vi "DisplayJson.vi"(11 "JSON String In":string="[{\"version\":\"1.0.0\",\"header\":{\"creationDate\":\"2022-06-03T00:00:00\",\"remarks\":\"\",\"serialNumber\":\"98172\",\"productNumber\":\"123021.1804\",\"productType\":\"PAA-9L\",\"pressureType\":2,\"productSeries\":\"9L\",\"compensatedTemperatureRange\":{\"min\":-10.0,\"max\":80.0,\"unit\":4},\"compensatedPressureRange\":{\"min\":0.0,\"max\":0.35,\"unit\":3},\"electricSupply\":{\"magnitude\":1.0,\"unit\":18},\"orderNumber\":9990266,\"orderPosition\":3,\"orderTargetDispatchDate\":\"2022-06-02T00:00:00+00:00\",\"customerName\":\"DemoData Inc.\",\"customerNumber\":12345678,\"customerOrderNumber\":\"Cust-9990266-123\",\"customerReferenceNumber\":\"\",\"customerProductT...") -> ()   [LabVIEW 2017] (continued)
\"unit\":4},\"supply\":{\"magnitude\":1.0,\"unit\":18}},\"raw\":{\"signal\":{\"magnitude\":16.118017703,\"unit\":22},\"bridgeResistance\":{\"magnitude\":3275.904706,\"unit\":28}},\"compensated\":{\"mathematicalModels\":{\"MM0123\":{\"pressure\":{\"output\":{\"magnitude\":0.0300104,\"unit\":3},\"error\":{\"magnitude\":0.00331228,\"unit\":7}},\"temperature\":{\"output\":{\"magnitude\":-10.8322,\"unit\":4},\"error\":{\"magnitude\":-0.10352768,\"unit\":4}}}}}},{\"reference\":\"F_12300_XX_0000098765\",\"environmentTarget\":{\"pressure\":{\"magnitude\":0.11,\"unit\":3},\"temperature\":{\"magnitude\":-10.0,\"unit\":4}},\"environment\":{\"pressure\":{\"magnitude\":0.110001,\"unit\":3},\"temperature\":{\"magnitude\":-10.7286,\"unit\":4},\"supply\":{\"magnitude\":1.0,\"unit\":18}},\"raw\":{\"signal\":{\"magnitude\":27.050815771,\"unit\":22},\"bridgeResistance\":{\"magnitude\":3271.7296615,\"unit\":28}},\"compensated\":{\"mathematicalModels\":{\"MM0123\":{\"pressure\":{\"output\":{\"magnitude\":0.109974,\"unit\":3},\"error\":{\"magnitude\":-0.0076162767,\"unit\":7}},\"temperature\":{\"output\":{\"magnitude\":-10.839,\"unit\":4},\"error\":{\"magnitude\":-0.11034124,\"unit\":4}}}}}},{\"reference\":\"F_12300_XX_0000098765\",\"environmentTarget\":{\"pressure\":{\"magnitude\":0.19,\"unit\":3},\"temperature\":{\"magnitude\":-10.0,\"unit\":4}},\"environment\":{\"pressure\":{\"magnitude\":0.190006,\"unit\":3},\"temperature\":{\"magnitude\":-10.7286,\"unit\":4},\"supply\":{\"magnitude\":1.0,\"unit\":18}},\"raw\":{\"signal\":{\"magnitude\":37.952972523,\"unit\":22},\"bridgeResistance\":{\"magnitude\":3267.7437326,\"unit\":28}},\"compensated\":{\"mathematicalModels\":{\"MM0123\":{\"pressure\":{\"output\":{\"magnitude\":0.190012,\"unit\":3},\"error\":{\"magnitude\":0.0016039999,\"unit\":7}},\"temperature\":{\"output\":{\"magnitude\":-10.8327,\"unit\":4},\"error\":{\"magnitude\":-0.10406948,\"unit\":4}}}}}},{\"reference\":\"F_12300_XX_0000098765\",\"environmentTarget\":{\"pressure\":{\"magnitude\":0.27,\"unit\":3},\"temperature\":{\"magnitude\":-10.0,\"unit\":4}},\"environment\":{\"pressure\":{\"magnitude\":0.270002,\"unit\":3},\"temperature\":{\"magnitude\":-10.7286,\"unit\":4},\"supply\":{\"magnitude\":1.0,\"unit\":18}},\"raw\":{\"signal\":{\"magnitude\":48.811226671,\"unit\":22},\"bridgeResistance\":{\"magnitude\":3263.8401462,\"unit\":28}},\"compensated\":{\"mathematicalModels\":{\"MM0123\":{\"pressure\":{\"output\":{\"magnitude\":0.270032,\"unit\":3},\"error\":{\"magnitude\":0.0086056558,\"unit\":7}},\"temperature\":{\"output\":{\"magnitude\":-10.8305,\"unit\":4},\"error\":{\"magnitude\":-0.10182691,\"unit\":4}}}}}},{\"reference\":\"F_12300_XX_0000098765\",\"environmentTarget\":{\"pressure\":{\"magnitude\":0.35,\"unit\":3},\"temperature\":{\"magnitude\":-10.0,\"unit\":4}},\"environment\":{\"pressure\":{\"magnitude\":0.350003,\"unit\":3},\"temperature\":{\"magnitude\":-10.7286,\"unit\":4},\"supply\":{\"magnitude\":1.0,\"unit\":18}},\"raw\":{\"signal\":{\"magnitude\":59.620114048,\"unit\":22},\"bridgeResistance\":{\"magnitude\":3259.9998996,\"unit\":28}},\"compensated\":{\"mathematicalModels\":{\"MM0123\":{\"pressure\":{\"output\":{\"magnitude\":0.349997,\"unit\":3},\"error\":{\"magnitude\":-0.0016426142,\"unit\":7}},\"temperature\":{\"output\":{\"magnitude\":-10.8357,\"unit\":4},\"error\":{\"magnitude\":-0.10710598,\"unit\":4}}}}}},{\"reference\":\"F_12300_XX_0000098765\",\"environmentTarget\":{\"pressure\":{\"magnitude\":0.03,\"unit\":3},\"temperature\":{\"magnitude\":0.0,\"unit\":4}},\"environment\":{\"pressure\":{\"magnitude\":0.0299997,\"unit\":3},\"temperature\":{\"magnitude\":-0.629962,\"unit\":4},\"supply\":{\"magnitude\":1.0,\"unit\":18}},\"raw\":{\"signal\":{\"magnitude\":16.568926387,\"unit\":22},\"bridgeResistance\":{\"magnitude\":3345.7360415,\"unit\":28}},\"compensated\":{\"mathematicalModels\":{\"MM0123\":{\"pressure\":{\"output\":{\"magnitude\":0.0300107,\"unit\":3},\"error\":{\"magnitude\":0.0031346511,\"unit\":7}},\"temperature\":{\"output\":{\"magnitude\":-0.744773,\"unit\":4},\"error\":{\"magnitude\":-0.11481098,\"unit\":4}}}}}},{\"reference\":\"F_12300_XX_0000098765\",\"environmentTarget\":{\"pressure\":{\"magnitude\":0.11,\"unit\":3},\"temperature\":{\"magnitude\":0.0,\"unit\":4}},\"environment\":{\"pressure\":{\"magnitude\":0.109998,\"unit\":3},\"temperature\":{\"magnitude\":-0.629962,\"unit\":4},\"supply\":{\"magnitude\":1.0,\"unit\":18}},\"raw\":{\"signal\":{\"magnitude\":27.469706317,\"unit\":22},\"bridgeResistance\":{\"magnitude\":3341.6261347,\"unit\":28}},\"compensated\":{\"mathematicalModels\":{\"MM0123\":{\"pressure\":{\"output\":{\"magnitude\":0.109974,\"unit\":3},\"error\":{\"magnitude\":-0.0069126471,\"unit\":7}},\"temperature\":{\"output\":{\"magnitude\":-0.743796,\"unit\":4},\"error\":{\"magnitude\":-0.11383453,\"unit\":4}}}}}},{\"reference\":\"F_12300_XX_0000098765\",\"environmentTarget\":{\"pressure\":{\"magnitude\":0.19,\"unit\":3},\"temperature\":{\"magnitude\":0.0,\"unit\":4}},\"environment\":{\"pressure\":{\"magnitude\":0.190003,\"unit\":3},\"temperature\":{\"magnitude\":-0.629962,\"unit\":4},\"supply\":{\"magnitude\":1.0,\"unit\":18}},\"raw\":{\"signal\":{\"magnitude\":38.339532672,\"unit\":22},\"bridgeResistance\":{\"magnitude\":3337.5825723,\"unit\":28}},\"compensated\":{\"mathematicalModels\":{\"MM0123\":{\"pressure\":{\"output\":{\"magnitude\":0.189998,\"unit\":3},\"error\":{\"magnitude\":-0.0014345835,\"unit\":7}},\"temperature\":{\"output\":{\"magnitude\":-0.746189,\"unit\":4},\"error\":{\"magnitude\":-0.11622639,\"unit\":4}}}}}},{\"reference\":\"F_12300_XX_0000098765\",\"environmentTarget\":{\"pressure\":{\"magnitude\":0.27,\"unit\":3},\"temperature\":{\"magnitude\":0.0,\"unit\":4}},\"environment\":{\"pressure\":{\"magnitude\":0.269999,\"unit\":3},\"temperature\":{\"magnitude\":-0.629962,\"unit\":4},\"supply\":{\"magnitude\":1.0,\"unit\":18}},\"raw\":{\"signal\":{\"magnitude\":49.167977875,\"unit\":22},\"bridgeResistance\":{\"magnitude\":3333.6130156,\"unit\":28}},\"compensated\":{\"mathematicalModels\":{\"MM0123\":{\"pressure\":{\"output\":{\"magnitude\":0.270007,\"unit\":3},\"error\":{\"magnitude\":0.0023560799,\"unit\":7}},\"temperature\":{\"output\":{\"magnitude\":-0.751685,\"unit\":4},\"error\":{\"magnitude\":-0.12172338,\"unit\":4}}}}}},{\"reference\":\"F_12300_XX_0000098765\",\"environmentTarget\":{\"pressure\":{\"magnitude\":0.35,\"unit\":3},\"temperature\":{\"magnitude\":0.0,\"unit\":4}},\"environment\":{\"pressure\":{\"magnitude\":0.350005,\"unit\":3},\"temperature\":{\"magnitude\":-0.629962,\"unit\":4},\"supply\":{\"magnitude\":1.0,\"unit\":18}},\"raw\":{\"signal\":{\"magnitude\":59.952257941,\"unit\":22},\"bridgeResistance\":{\"magnitude\":3329.770464,\"unit\":28}},\"compensated\":{\"mathematicalModels\":{\"MM0123\":{\"pressure\":{\"output\":{\"magnitude\":0.349979,\"unit\":3},\"error\":{\"magnitude\":-0.0073028693,\"unit\":7}},\"temperature\":{\"output\":{\"magnitude\":-0.753307,\"unit\":4},\"error\":{\"magnitude\":-0.12334541,\"unit\":4}}}}}},{\"reference\":\"F_12300_XX_0000098765\",\"environmentTarget\":{\"pressure\":{\"magnitude\":0.03,\"unit\":3},\"temperature\":{\"magnitude\":20.0,\"unit\":4}},\"environment\":{\"pressure\":{\"magnitude\":0.0300032,\"unit\":3},\"temperature\":{\"magnitude\":19.5509,\"unit\":4},\"supply\":{\"magnitude\":1.0,\"unit\":18}},\"raw\":{\"signal\":{\"magnitude\":17.508789568,\"unit\":22},\"bridgeResistance\":{\"magnitude\":3502.485602,\"unit\":28}},\"compensated\":{\"mathematicalModels\":{\"MM0123\":{\"pressure\":{\"output\":{\"magnitude\":0.0300153,\"unit\":3},\"error\":{\"magnitude\":0.0034436329,\"unit\":7}},\"temperature\":{\"output\":{\"magnitude\":19.5499,\"unit\":4},\"error\":{\"magnitude\":-0.00093978929,\"unit\":4}}}}}},{\"reference\":\"F_12300_XX_0000098765\",\"environmentTarget\":{\"pressure\":{\"magnitude\":0.11,\"unit\":3},\"temperature\":{\"magnitude\":20.0,\"unit\":4}},\"environment\":{\"pressure\":{\"magnitude\":0.109996,\"unit\":3},\"temperature\":{\"magnitude\":19.5509,\"unit\":4},\"supply\":{\"magnitude\":1.0,\"unit\":18}},\"raw\":{\"signal\":{\"magnitude\":28.398706548,\"unit\":22},\"bridgeResistance\":{\"magnitude\":3498.325108,\"unit\":28}},\"compensated\":{\"mathematicalModels\":{\"MM0123\":{\"pressure\":{\"output\":{\"magnitude\":0.109974,\"unit\":3},\"error\":{\"magnitude\":-0.0063104891,\"unit\":7}},\"temperature\":{\"output\":{\"magnitude\":19.5428,\"unit\":4},\"error\":{\"magnitude\":-0.0081190802,\"unit\":4}}}}}},{\"reference\":\"F_12300_XX_0000098765\",\"environmentTarget\":{\"pressure\":{\"magnitude\":0.19,\"unit\":3},\"temperature\":{\"magnitude\":20.0,\"unit\":4}},\"environment\":{\"pressure\":{\"magnitude\":0.189992,\"unit\":3},\"temperature\":{\"magnitude\":19.5509,\"unit\":4},\"supply\":{\"magnitude\":1.0,\"unit\":18}},\"raw\":{\"signal\":{\"magnitude\":39.263123148,\"unit\":22},\"bridgeResistance\":{\"magnitude\":3494.3052236,\"unit\":28}},\"compensated\":{\"mathematicalModels\":{\"MM0123\":{\"pressure\":{\"output\":{\"magnitude\":0.190003,\"unit\":3},\"error\":{\"magnitude\":0.0031341282,\"unit\":7}},\"temperature\":{\"output\":{\"magnitude\":19.5435,\"unit\":4},\"error\":{\"magnitude\":-0.0073409516,\"unit\":4}}}}}},{\"reference\":\"F_12300_XX_0000098765\",\"environmentTarget\":{\"pressure\":{\"magnitude\":0.27,\"unit\":3},\"temperature\":{\"magnitude\":20.0,\"unit\":4}},\"environment\":{\"pressure\":{\"magnitude\":0.269993,\"unit\":3},\"temperature\":{\"magnitude\":19.5509,\"unit\":4},\"supply\":{\"magnitude\":1.0,\"unit\":18}},\"raw\":{\"signal\":{\"magnitude\":50.090798002,\"unit\":22},\"bridgeResistance\":{\"magnitude\":3490.3161774,\"unit\":28}},\"compensated\":{\"mathematicalModels\":{\"MM0123\":{\"pressure\":{\"output\":{\"magnitude\":0.270025,\"unit\":3},\"error\":{\"magnitude\":0.0091306696,\"unit\":7}},\"temperature\":{\"output\":{\"magnitude\":19.5384,\"unit\":4},\"error\":{\"magnitude\":-0.012497416,\"unit\":4}}}}}},{\"reference\":\"F_12300_XX_0000098765\",\"environmentTarget\":{\"pressure\":{\"magnitude\":0.35,\"unit\":3},\"temperature\":{\"magnitude\":20.0,\"unit\":4}},\"environment\":{\"pressure\":{\"magnitude\":0.350012,\"unit\":3},\"temperature\":{\"magnitude\":19.5509,\"unit\":4},\"supply\":{\"magnitude\":1.0,\"unit\":18}},\"raw\":{\"signal\":{\"magnitude\":60.879181622,\"unit\":22},\"bridgeResistance\":{\"magnitude\":3486.4490777,\"unit\":28}},\"compensated\":{\"mathematicalModels\":{\"MM0123\":{\"pressure\":{\"output\":{\"magnitude\":0.350017,\"unit\":3},\"error\":{\"magnitude\":0.0013342798,\"unit\":7}},\"temperature\":{\"output\":{\"magnitude\":19.5381,\"unit\":4},\"error\":{\"magnitude\":-0.012768281,\"unit\":4}}}}}},{\"reference\":\"F_12300_XX_0000098765\",\"environmentTarget\":{\"pressure\":{\"magnitude\":0.03,\"unit\":3},\"temperature\":{\"magnitude\":40.0,\"unit\":4}},\"environment\":{\"pressure\":{\"magnitude\":0.0299978,\"unit\":3},\"temperature\":{\"magnitude\":39.7284,\"unit\":4},\"supply\":{\"magnitude\":1.0,\"unit\":18}},\"raw\":{\"signal\":{\"magnitude\":18.512052925,\"unit\":22},\"bridgeResistance\":{\"magnitude\":3678.2402787,\"unit\":28}},\"compensated\":{\"mathematicalModels\":{\"MM0123\":{\"pressure\":{\"output\":{\"magnitude\":0.0300125,\"unit\":3},\"error\":{\"magnitude\":0.0041964975,\"unit\":7}},\"temperature\":{\"output\":{\"magnitude\":39.7197,\"unit\":4},\"error\":{\"magnitude\":-0.0086930497,\"unit\":4}}}}}},{\"reference\":\"F_12300_XX_0000098765\",\"environmentTarget\":{\"pressure\":{\"magnitude\":0.11,\"unit\":3},\"temperature\":{\"magnitude\":40.0,\"unit\":4}},\"environment\":{\"pressure\":{\"magnitude\":0.110012,\"unit\":3},\"temperature\":{\"magnitude\":39.7284,\"unit\":4},\"supply\":{\"magnitude\":1.0,\"unit\":18}},\"raw\":{\"signal\":{\"magnitude\":29.451517412,\"unit\":22},\"bridgeResistance\":{\"magnitude\":3674.1165555,\"unit\":28}},\"compensated\":{\"mathematicalModels\":{\"MM0123\":{\"pressure\":{\"output\":{\"magnitude\":0.109976,\"unit\":3},\"error\":{\"magnitude\":-0.01022075,\"unit\":7}},\"temperature\":{\"output\":{\"magnitude\":39.7193,\"unit\":4},\"error\":{\"magnitude\":-0.0091078646,\"unit\":4}}}}}},{\"reference\":\"F_12300_XX_0000098765\",\"environmentTarget\":{\"pressure\":{\"magnitude\":0.19,\"unit\":3},\"temperature\":{\"magnitude\":40.0,\"unit\":4}},\"environment\":{\"pressure\":{\"magnitude\":0.190003,\"unit\":3},\"temperature\":{\"magnitude\":39.7284,\"unit\":4},\"supply\":{\"magnitude\":1.0,\"unit\":18}},\"raw\":{\"signal\":{\"magnitude\":40.368344408,\"unit\":22},\"bridgeResistance\":{\"magnitude\":3670.043361,\"unit\":28}},\"compensated\":{\"mathematicalModels\":{\"MM0123\":{\"pressure\":{\"output\":{\"magnitude\":0.190005,\"unit\":3},\"error\":{\"magnitude\":0.00066025861,\"unit\":7}},\"temperature\":{\"output\":{\"magnitude\":39.7172,\"unit\":4},\"error\":{\"magnitude\":-0.01127367,\"unit\":4}}}}}},{\"reference\":\"F_12300_XX_0000098765\",\"environmentTarget\":{\"pressure\":{\"magnitude\":0.27,\"unit\":3},\"temperature\":{\"magnitude\":40.0,\"unit\":4}},\"environment\":{\"pressure\":{\"magnitude\":0.269991,\"unit\":3},\"temperature\":{\"magnitude\":39.7284,\"unit\":4},\"supply\":{\"magnitude\":1.0,\"unit\":18}},\"raw\":{\"signal\":{\"magnitude\":51.249896616,\"unit\":22},\"bridgeResistance\":{\"magnitude\":3666.0556113,\"unit\":28}},\"compensated\":{\"mathematicalModels\":{\"MM0123\":{\"pressure\":{\"output\":{\"magnitude\":0.270006,\"unit\":3},\"error\":{\"magnitude\":0.0043130135,\"unit\":7}},\"temperature\":{\"output\":{\"magnitude\":39.7168,\"unit\":4},\"error\":{\"magnitude\":-0.011660585,\"unit\":4}}}}}},{\"reference\":\"F_12300_XX_0000098765\",\"environmentTarget\":{\"pressure\":{\"magnitude\":0.35,\"unit\":3},\"temperature\":{\"magnitude\":40.0,\"unit\":4}},\"environment\":{\"pressure\":{\"magnitude\":0.350007,\"unit\":3},\"temperature\":{\"magnitude\":39.7284,\"unit\":4},\"supply\":{\"magnitude\":1.0,\"unit\":18}},\"raw\":{\"signal\":{\"magnitude\":62.096595353,\"unit\":22},\"bridgeResistance\":{\"magnitude\":3662.1121149,\"unit\":28}},\"compensated\":{\"mathematicalModels\":{\"MM0123\":{\"pressure\":{\"output\":{\"magnitude\":0.349984,\"unit\":3},\"error\":{\"magnitude\":-0.006660769,\"unit\":7}},\"temperature\":{\"output\":{\"magnitude\":39.7132,\"unit\":4},\"error\":{\"magnitude\":-0.015214193,\"unit\":4}}}}}},{\"reference\":\"F_12300_XX_0000098765\",\"environmentTarget\":{\"pressure\":{\"magnitude\":0.03,\"unit\":3},\"temperature\":{\"magnitude\":60.0,\"unit\":4}},\"environment\":{\"pressure\":{\"magnitude\":0.0299911,\"unit\":3},\"temperature\":{\"magnitude\":59.8651,\"unit\":4},\"supply\":{\"magnitude\":1.0,\"unit\":18}},\"raw\":{\"signal\":{\"magnitude\":19.614878521,\"unit\":22},\"bridgeResistance\":{\"magnitude\":3870.4360415,\"unit\":28}},\"compensated\":{\"mathematicalModels\":{\"MM0123\":{\"pressure\":{\"output\":{\"magnitude\":0.0300063,\"unit\":3},\"error\":{\"magnitude\":0.0043445952,\"unit\":7}},\"temperature\":{\"output\":{\"magnitude\":59.9283,\"unit\":4},\"error\":{\"magnitude\":0.063173095,\"unit\":4}}}}}},{\"reference\":\"F_12300_XX_0000098765\",\"environmentTarget\":{\"pressure\":{\"magnitude\":0.11,\"unit\":3},\"temperature\":{\"magnitude\":60.0,\"unit\":4}},\"environment\":{\"pressure\":{\"magnitude\":0.11,\"unit\":3},\"temperature\":{\"magnitude\":59.8651,\"unit\":4},\"supply\":{\"magnitude\":1.0,\"unit\":18}},\"raw\":{\"signal\":{\"magnitude\":30.638429504,\"unit\":22},\"bridgeResistance\":{\"magnitude\":3866.2610003,\"unit\":28}},\"compensated\":{\"mathematicalModels\":{\"MM0123\":{\"pressure\":{\"output\":{\"magnitude\":0.10997,\"unit\":3},\"error\":{\"magnitude\":-0.0086978031,\"unit\":7}},\"temperature\":{\"output\":{\"magnitude\":59.9299,\"unit\":4},\"error\":{\"magnitude\":0.06477835,\"unit\":4}}}}}},{\"reference\":\"F_12300_XX_0000098765\",\"environmentTarget\":{\"pressure\":{\"magnitude\":0.19,\"unit\":3},\"temperature\":{\"magnitude\":60.0,\"unit\":4}},\"environment\":{\"pressure\":{\"magnitude\":0.189995,\"unit\":3},\"temperature\":{\"magnitude\":59.8651,\"unit\":4},\"supply\":{\"magnitude\":1.0,\"unit\":18}},\"raw\":{\"signal\":{\"magnitude\":41.64509949,\"unit\":22},\"bridgeResistance\":{\"magnitude\":3862.1495484,\"unit\":28}},\"compensated\":{\"mathematicalModels\":{\"MM0123\":{\"pressure\":{\"output\":{\"magnitude\":0.190003,\"unit\":3},\"error\":{\"magnitude\":0.00236892,\"unit\":7}},\"temperature\":{\"output\":{\"magnitude\":59.9328,\"unit\":4},\"error\":{\"magnitude\":0.067646361,\"unit\":4}}}}}},{\"reference\":\"F_12300_XX_0000098765\",\"environmentTarget\":{\"pressure\":{\"magnitude\":0.27,\"unit\":3},\"temperature\":{\"magnitude\":60.0,\"unit\":4}},\"environment\":{\"pressure\":{\"magnitude\":0.270008,\"unit\":3},\"temperature\":{\"magnitude\":59.8651,\"unit\":4},\"supply\":{\"magnitude\":1.0,\"unit\":18}},\"raw\":{\"signal\":{\"magnitude\":52.624237436,\"unit\":22},\"bridgeResistance\":{\"magnitude\":3858.0534892,\"unit\":28}},\"compensated\":{\"mathematicalModels\":{\"MM0123\":{\"pressure\":{\"output\":{\"magnitude\":0.270034,\"unit\":3},\"error\":{\"magnitude\":0.007359755,\"unit\":7}},\"temperature\":{\"output\":{\"magnitude\":59.9315,\"unit\":4},\"error\":{\"magnitude\":0.06640627,\"unit\":4}}}}}},{\"reference\":\"F_12300_XX_0000098765\",\"environmentTarget\":{\"pressure\":{\"magnitude\":0.35,\"unit\":3},\"temperature\":{\"magnitude\":60.0,\"unit\":4}},\"environment\":{\"pressure\":{\"magnitude\":0.349996,\"unit\":3},\"temperature\":{\"magnitude\":59.8651,\"unit\":4},\"supply\":{\"magnitude\":1.0,\"unit\":18}},\"raw\":{\"signal\":{\"magnitude\":63.566437591,\"unit\":22},\"bridgeResistance\":{\"magnitude\":3854.0794025,\"unit\":28}},\"compensated\":{\"mathematicalModels\":{\"MM0123\":{\"pressure\":{\"output\":{\"magnitude\":0.349987,\"unit\":3},\"error\":{\"magnitude\":-0.002465495,\"unit\":7}},\"temperature\":{\"output\":{\"magnitude\":59.9366,\"unit\":4},\"error\":{\"magnitude\":0.071417544,\"unit\":4}}}}}},{\"reference\":\"F_12300_XX_0000098765\",\"environmentTarget\":{\"pressure\":{\"magnitude\":0.03,\"unit\":3},\"temperature\":{\"magnitude\":80.0,\"unit\":4}},\"environment\":{\"pressure\":{\"magnitude\":0.0300073,\"unit\":3},\"temperature\":{\"magnitude\":79.9513,\"unit\":4},\"supply\":{\"magnitude\":1.0,\"unit\":18}},\"raw\":{\"signal\":{\"magnitude\":20.849559966,\"unit\":22},\"bridgeResistance\":{\"magnitude\":4077.7682758,\"unit\":28}},\"compensated\":{\"mathematicalModels\":{\"MM0123\":{\"pressure\":{\"output\":{\"magnitude\":0.0300251,\"unit\":3},\"error\":{\"magnitude\":0.0050764202,\"unit\":7}},\"temperature\":{\"output\":{\"magnitude\":80.0453,\"unit\":4},\"error\":{\"magnitude\":0.093925947,\"unit\":4}}}}}},{\"reference\":\"F_12300_XX_0000098765\",\"environmentTarget\":{\"pressure\":{\"magnitude\":0.11,\"unit\":3},\"temperature\":{\"magnitude\":80.0,\"unit\":4}},\"environment\":{\"pressure\":{\"magnitude\":0.11,\"unit\":3},\"temperature\":{\"magnitude\":79.9513,\"unit\":4},\"supply\":{\"magnitude\":1.0,\"unit\":18}},\"raw\":{\"signal\":{\"magnitude\":31.983210178,\"unit\":22},\"bridgeResistance\":{\"magnitude\":4073.5137666,\"unit\":28}},\"compensated\":{\"mathematicalModels\":{\"MM0123\":{\"pressure\":{\"output\":{\"magnitude\":0.109962,\"unit\":3},\"error\":{\"magnitude\":-0.010869658,\"unit\":7}},\"temperature\":{\"output\":{\"magnitude\":80.0467,\"unit\":4},\"error\":{\"magnitude\":0.095334982,\"unit\":4}}}}}},{\"reference\":\"F_12300_XX_0000098765\",\"environmentTarget\":{\"pressure\":{\"magnitude\":0.19,\"unit\":3},\"temperature\":{\"magnitude\":80.0,\"unit\":4}},\"environment\":{\"pressure\":{\"magnitude\":0.190006,\"unit\":3},\"temperature\":{\"magnitude\":79.9513,\"unit\":4},\"supply\":{\"magnitude\":1.0,\"unit\":18}},\"raw\":{\"signal\":{\"magnitude\":43.110258467,\"unit\":22},\"bridgeResistance\":{\"magnitude\":4069.3635428,\"unit\":28}},\"compensated\":{\"mathematicalModels\":{\"MM0123\":{\"pressure\":{\"output\":{\"magnitude\":0.19001,\"unit\":3},\"error\":{\"magnitude\":0.0012686748,\"unit\":7}},\"temperature\":{\"output\":{\"magnitude\":80.0543,\"unit\":4},\"error\":{\"magnitude\":0.10295016,\"unit\":4}}}}}},{\"reference\":\"F_12300_XX_0000098765\",\"environmentTarget\":{\"pressure\":{\"magnitude\":0.27,\"unit\":3},\"temperature\":{\"magnitude\":80.0,\"unit\":4}},\"environment\":{\"pressure\":{\"magnitude\":0.270003,\"unit\":3},\"temperature\":{\"magnitude\":79.9513,\"unit\":4},\"supply\":{\"magnitude\":1.0,\"unit\":18}},\"raw\":{\"signal\":{\"magnitude\":54.211299756,\"unit\":22},\"bridgeResistance\":{\"magnitude\":4065.2570498,\"unit\":28}},\"compensated\":{\"mathematicalModels\":{\"MM0123\":{\"pressure\":{\"output\":{\"magnitude\":0.270034,\"unit\":3},\"error\":{\"magnitude\":0.0089724607,\"unit\":7}},\"temperature\":{\"output\":{\"magnitude\":80.0619,\"unit\":4},\"error\":{\"magnitude\":0.11056394,\"unit\":4}}}}}},{\"reference\":\"F_12300_XX_0000098765\",\"environmentTarget\":{\"pressure\":{\"magnitude\":0.35,\"unit\":3},\"temperature\":{\"magnitude\":80.0,\"unit\":4}},\"environment\":{\"pressure\":{\"magnitude\":0.350007,\"unit\":3},\"temperature\":{\"magnitude\":79.9513,\"unit\":4},\"supply\":{\"magnitude\":1.0,\"unit\":18}},\"raw\":{\"signal\":{\"magnitude\":65.27989423,\"unit\":22},\"bridgeResistance\":{\"magnitude\":4061.1476956,\"unit\":28}},\"compensated\":{\"mathematicalModels\":{\"MM0123\":{\"pressure\":{\"output\":{\"magnitude\":0.34999,\"unit\":3},\"error\":{\"magnitude\":-0.0047163655,\"unit\":7}},\"temperature\":{\"output\":{\"magnitude\":80.0651,\"unit\":4},\"error\":{\"magnitude\":0.11370689,\"unit\":4}}}}}}]},{\"version\":\"1.0.0\",\"header\":{\"creationDate\":\"2022-06-03T00:00:00\",\"remarks\":\"\",\"serialNumber\":\"98013\",\"productNumber\":\"123021.1804\",\"productType\":\"PAA-9L\",\"pressureType\":2,\"productSeries\":\"9L\",\"compensatedTemperatureRange\":{\"min\":-10.0,\"max\":80.0,\"unit\":4},\"compensatedPressureRange\":{\"min\":0.0,\"max\":0.35,\"unit\":3},\"electricSupply\":{\"magnitude\":1.0,\"unit\":18},\"orderNumber\":9990266,\"orderPosition\":3,\"orderTargetDispatchDate\":\"2022-06-02T00:00:00+00:00\",\"customerName\":\"DemoData Inc.\",\"customerNumber\":12345678,\"customerOrderNumber\":\"Cust-9990266-123\",\"customerReferenceNumber\":\"\",\"customerProductType\":\"123021-1804 Rev.AA\"},\"compensationMethods\":{\"mathematicalModels\":{\"MM0123\":{\"modelType\":\"MM0123\",\"productNumber\":\"000000.0000\",\"compensatedTemperatureRange\":{\"min\":-10.0,\"max\":80.0,\"unit\":4},\"compensatedPressureRange\":{\"min\":0.0,\"max\":0.35,\"unit\":3},\"electricSupply\":{\"magnitude\":1.0,\"unit\":18},\"parts\":{\"pressure\":{\"inputs\":[\"Sig\",\"R\"],\"output\":\"P\",\"description\":\"P = f(Sig,R)\",\"coefficients\":[[4.4457335518,-0.00454206635857,1.72804105458E-06,-2.94337525476E-10,1.87900124337E-14],[-0.137303639989,0.000147633012571,-5.67112931747E-08,9.67929265896E-12,-6.20473324595E-16],[7.01661893009E-05,-5.36472642526E-08,1.42800617063E-11,-1.37323280897E-15,1.72584035529E-20]]},\"temperature\":{\"inputs\":[\"R\",\"Sig\"],\"output\":\"T\",\"description\":\"T = f(R,Sig)\",\"coefficients\":[[-7816.11608154,-3.51493452401,0.0109404942103],[7.67845932211,0.00490503550809,-1.28219864107E-05],[-0.00289502810298,-2.3662581924E-06,5.45467377186E-09],[4.94755555462E-07,4.86516563214E-10,-1.00829275973E-12],[-3.1915287397E-11,-3.64996092282E-14,6.87014771591E-17]]}}}}},\"measurements\":[{\"reference\":\"F_12300_XX_0000098765\",\"environmentTarget\":{\"pressure\":{\"magnitude\":0.03,\"unit\":3},\"temperature\":{\"magnitude\":-10.0,\"unit\":4}},\"environment\":{\"pressure\":{\"magnitude\":0.0300065,\"unit\":3},\"temperature\":{\"magnitude\":-10.7286,\"unit\":4},\"supply\":{\"magnitude\":1.0,\"unit\":18}},\"raw\":{\"signal\":{\"magnitude\":15.664929263,\"unit\":22},\"bridgeResistance\":{\"magnitude\":3280.926027,\"unit\":28}},\"compensated\":{\"mathematicalModels\":{\"MM0123\":{\"pressure\":{\"output\":{\"magnitude\":0.0300208,\"unit\":3},\"error\":{\"magnitude\":0.004079608,\"unit\":7}},\"temperature\":{\"output\":{\"magnitude\":-10.8433,\"unit\":4},\"error\":{\"magnitude\":-0.11462482,\"unit\":4}}}}}},{\"reference\":\"F_12300_XX_0000098765\",\"environmentTarget\":{\"pressure\":{\"magnitude\":0.11,\"unit\":3},\"temperature\":{\"magnitude\":-10.0,\"unit\":4}},\"environment\":{\"pressure\":{\"magnitude\":0.11001,\"unit\":3},\"temperature\":{\"magnitude\":-10.7286,\"unit\":4},\"supply\":{\"magnitude\":1.0,\"unit\":18}},\"raw\":{\"signal\":{\"magnitude\":27.72520271,\"unit\":22},\"bridgeResistance\":{\"magnitude\":3276.2530208,\"unit\":28}},\"compensated\":{\"mathematicalModels\":{\"MM0123\":{\"pressure\":{\"output\":{\"magnitude\":0.109975,\"unit\":3},\"error\":{\"magnitude\":-0.010067232,\"unit\":7}},\"temperature\":{\"output\":{\"magnitude\":-10.8505,\"unit\":4},\"error\":{\"magnitude\":-0.1218544,\"unit\":4}}}}}},{\"reference\":\"F_12300_XX_0000098765\",\"environmentTarget\":{\"pressure\":{\"magnitude\":0.19,\"unit\":3},\"temperature\":{\"magnitude\":-10.0,\"unit\":4}},\"environment\":{\"pressure\":{\"magnitude\":0.190004,\"unit\":3},\"temperature\":{\"magnitude\":-10.7286,\"unit\":4},\"supply\":{\"magnitude\":1.0,\"unit\":18}},\"raw\":{\"signal\":{\"magnitude\":39.744559453,\"unit\":22},\"bridgeResistance\":{\"magnitude\":3271.7868626,\"unit\":28}},\"compensated\":{\"mathematicalModels\":{\"MM0123\":{\"pressure\":{\"output\":{\"magnitude\":0.190012,\"unit\":3},\"error\":{\"magnitude\":0.0022741612,\"unit\":7}},\"temperature\":{\"output\":{\"magnitude\":-10.8436,\"unit\":4},\"error\":{\"magnitude\":-0.11501229,\"unit\":4}}}}}},{\"reference\":\"F_12300_XX_0000098765\",\"environmentTarget\":{\"pressure\":{\"magnitude\":0.27,\"unit\":3},\"temperature\":{\"magnitude\":-10.0,\"unit\":4}},\"environment\":{\"pressure\":{\"magnitude\":0.27,\"unit\":3},\"temperature\":{\"magnitude\":-10.7286,\"unit\":4},\"supply\":{\"magnitude\":1.0,\"unit\":18}},\"raw\":{\"signal\":{\"magnitude\":51.707176409,\"unit\":22},\"bridgeResistance\":{\"magnitude\":3267.3904934,\"unit\":28}},\"compensated\":{\"mathematicalModels\":{\"MM0123\":{\"pressure\":{\"output\":{\"magnitude\":0.270035,\"unit\":3},\"error\":{\"magnitude\":0.010031402,\"unit\":7}},\"temperature\":{\"output\":{\"magnitude\":-10.8443,\"unit\":4},\"error\":{\"magnitude\":-0.11567292,\"unit\":4}}}}}},{\"reference\":\"F_12300_XX_0000098765\",\"environmentTarget\":{\"pressure\":{\"magnitude\":0.35,\"unit\":3},\"temperature\":{\"magnitude\":-10.0,\"unit\":4}},\"environment\":{\"pressure\":{\"magnitude\":0.35,\"unit\":3},\"temperature\":{\"magnitude\":-10.7286,\"unit\":4},\"supply\":{\"magnitude\":1.0,\"unit\":18}},\"raw\":{\"signal\":{\"magnitude\":63.605422182,\"unit\":22},\"bridgeResistance\":{\"magnitude\":3263.0911906,\"unit\":28}},\"compensated\":{\"mathematicalModels\":{\"MM0123\":{\"pressure\":{\"output\":{\"magnitude\":0.349993,\"unit\":3},\"error\":{\"magnitude\":-0.0021344751,\"unit\":7}},\"temperature\":{\"output\":{\"magnitude\":-10.849,\"unit\":4},\"error\":{\"magnitude\":-0.12032792,\"unit\":4}}}}}},{\"reference\":\"F_12300_XX_0000098765\",\"environmentTarget\":{\"pressure\":{\"magnitude\":0.03,\"unit\":3},\"temperature\":{\"magnitude\":0.0,\"unit\":4}},\"environment\":{\"pressure\":{\"magnitude\":0.0300019,\"unit\":3},\"temperature\":{\"magnitude\":-0.629962,\"unit\":4},\"supply\":{\"magnitude\":1.0,\"unit\":18}},\"raw\":{\"signal\":{\"magnitude\":16.151547564,\"unit\":22},\"bridgeResistance\":{\"magnitude\":3350.9437776,\"unit\":28}},\"compensated\":{\"mathematicalModels\":{\"MM0123\":{\"pressure\":{\"output\":{\"magnitude\":0.0300165,\"unit\":3},\"error\":{\"magnitude\":0.0041851521,\"unit\":7}},\"temperature\":{\"output\":{\"magnitude\":-0.752132,\"unit\":4},\"error\":{\"magnitude\":-0.12217046,\"unit\":4}}}}}},{\"reference\":\"F_12300_XX_0000098765\",\"environmentTarget\":{\"pressure\":{\"magnitude\":0.11,\"unit\":3},\"temperature\":{\"magnitude\":0.0,\"unit\":4}},\"environment\":{\"pressure\":{\"magnitude\":0.110001,\"unit\":3},\"temperature\":{\"magnitude\":-0.629962,\"unit\":4},\"supply\":{\"magnitude\":1.0,\"unit\":18}},\"raw\":{\"signal\":{\"magnitude\":28.178004953,\"unit\":22},\"bridgeResistance\":{\"magnitude\":3346.3205845,\"unit\":28}},\"compensated\":{\"mathematicalModels\":{\"MM0123\":{\"pressure\":{\"output\":{\"magnitude\":0.109968,\"unit\":3},\"error\":{\"magnitude\":-0.0093451802,\"unit\":7}},\"temperature\":{\"output\":{\"magnitude\":-0.752551,\"unit\":4},\"error\":{\"magnitude\":-0.12258946,\"unit\":4}}}}}},{\"reference\":\"F_12300_XX_0000098765\",\"environmentTarget\":{\"pressure\":{\"magnitude\":0.19,\"unit\":3},\"temperature\":{\"magnitude\":0.0,\"unit\":4}},\"environment\":{\"pressure\":{\"magnitude\":0.190005,\"unit\":3},\"temperature\":{\"magnitude\":-0.629962,\"unit\":4},\"supply\":{\"magnitude\":1.0,\"unit\":18}},\"raw\":{\"signal\":{\"magnitude\":40.165142254,\"unit\":22},\"bridgeResistance\":{\"magnitude\":3341.7893432,\"unit\":28}},\"compensated\":{\"mathematicalModels\":{\"MM0123\":{\"pressure\":{\"output\":{\"magnitude\":0.190001,\"unit\":3},\"error\":{\"magnitude\":-0.0012387905,\"unit\":7}},\"temperature\":{\"output\":{\"magnitude\":-0.754961,\"unit\":4},\"error\":{\"magnitude\":-0.12499915,\"unit\":4}}}}}},{\"reference\":\"F_12300_XX_0000098765\",\"environmentTarget\":{\"pressure\":{\"magnitude\":0.27,\"unit\":3},\"temperature\":{\"magnitude\":0.0,\"unit\":4}},\"environment\":{\"pressure\":{\"magnitude\":0.269999,\"unit\":3},\"temperature\":{\"magnitude\":-0.629962,\"unit\":4},\"supply\":{\"magnitude\":1.0,\"unit\":18}},\"raw\":{\"signal\":{\"magnitude\":52.097670281,\"unit\":22},\"bridgeResistance\":{\"magnitude\":3337.3400559,\"unit\":28}},\"compensated\":{\"mathematicalModels\":{\"MM0123\":{\"pressure\":{\"output\":{\"magnitude\":0.270013,\"unit\":3},\"error\":{\"magnitude\":0.0040281493,\"unit\":7}},\"temperature\":{\"output\":{\"magnitude\":-0.761348,\"unit\":4},\"error\":{\"magnitude\":-0.13138577,\"unit\":4}}}}}},{\"reference\":\"F_12300_XX_0000098765\",\"environmentTarget\":{\"pressure\":{\"magnitude\":0.35,\"unit\":3},\"temperature\":{\"magnitude\":0.0,\"unit\":4}},\"environment\":{\"pressure\":{\"magnitude\":0.35,\"unit\":3},\"temperature\":{\"magnitude\":-0.629962,\"unit\":4},\"supply\":{\"magnitude\":1.0,\"unit\":18}},\"raw\":{\"signal\":{\"magnitude\":63.970587795,\"unit\":22},\"bridgeResistance\":{\"magnitude\":3333.0370698,\"unit\":28}},\"compensated\":{\"mathematicalModels\":{\"MM0123\":{\"pressure\":{\"output\":{\"magnitude\":0.34997,\"unit\":3},\"error\":{\"magnitude\":-0.0086490475,\"unit\":7}},\"temperature\":{\"output\":{\"magnitude\":-0.763639,\"unit\":4},\"error\":{\"magnitude\":-0.1336774,\"unit\":4}}}}}},{\"reference\":\"F_12300_XX_0000098765\",\"environmentTarget\":{\"pressure\":{\"magnitude\":0.03,\"unit\":3},\"temperature\":{\"magnitude\":20.0,\"unit\":4}},\"environment\":{\"pressure\":{\"magnitude\":0.0299994,\"unit\":3},\"temperature\":{\"magnitude\":19.5509,\"unit\":4},\"supply\":{\"magnitude\":1.0,\"unit\":18}},\"raw\":{\"signal\":{\"magnitude\":17.163422,\"unit\":22},\"bridgeResistance\":{\"magnitude\":3508.0606507,\"unit\":28}},\"compensated\":{\"mathematicalModels\":{\"MM0123\":{\"pressure\":{\"output\":{\"magnitude\":0.0300147,\"unit\":3},\"error\":{\"magnitude\":0.0043735365,\"unit\":7}},\"temperature\":{\"output\":{\"magnitude\":19.5459,\"unit\":4},\"error\":{\"magnitude\":-0.0049851929,\"unit\":4}}}}}},{\"reference\":\"F_12300_XX_0000098765\",\"environmentTarget\":{\"pressure\":{\"magnitude\":0.11,\"unit\":3},\"temperature\":{\"magnitude\":20.0,\"unit\":4}},\"environment\":{\"pressure\":{\"magnitude\":0.109996,\"unit\":3},\"temperature\":{\"magnitude\":19.5509,\"unit\":4},\"supply\":{\"magnitude\":1.0,\"unit\":18}},\"raw\":{\"signal\":{\"magnitude\":29.181982448,\"unit\":22},\"bridgeResistance\":{\"magnitude\":3503.4104398,\"unit\":28}},\"compensated\":{\"mathematicalModels\":{\"MM0123\":{\"pressure\":{\"output\":{\"magnitude\":0.109967,\"unit\":3},\"error\":{\"magnitude\":-0.0081447182,\"unit\":7}},\"temperature\":{\"output\":{\"magnitude\":19.5405,\"unit\":4},\"error\":{\"magnitude\":-0.010344002,\"unit\":4}}}}}},{\"reference\":\"F_12300_XX_0000098765\",\"environmentTarget\":{\"pressure\":{\"magnitude\":0.19,\"unit\":3},\"temperature\":{\"magnitude\":20.0,\"unit\":4}},\"environment\":{\"pressure\":{\"magnitude\":0.189989,\"unit\":3},\"temperature\":{\"magnitude\":19.5509,\"unit\":4},\"supply\":{\"magnitude\":1.0,\"unit\":18}},\"raw\":{\"signal\":{\"magnitude\":41.166218036,\"unit\":22},\"bridgeResistance\":{\"magnitude\":3498.8781748,\"unit\":28}},\"compensated\":{\"mathematicalModels\":{\"MM0123\":{\"pressure\":{\"output\":{\"magnitude\":0.189999,\"unit\":3},\"error\":{\"magnitude\":0.0029958939,\"unit\":7}},\"temperature\":{\"output\":{\"magnitude\":19.5389,\"unit\":4},\"error\":{\"magnitude\":-0.011984444,\"unit\":4}}}}}},{\"reference\":\"F_12300_XX_0000098765\",\"environmentTarget\":{\"pressure\":{\"magnitude\":0.27,\"unit\":3},\"temperature\":{\"magnitude\":20.0,\"unit\":4}},\"environment\":{\"pressure\":{\"magnitude\":0.269991,\"unit\":3},\"temperature\":{\"magnitude\":19.5509,\"unit\":4},\"supply\":{\"magnitude\":1.0,\"unit\":18}},\"raw\":{\"signal\":{\"magnitude\":53.103928296,\"unit\":22},\"bridgeResistance\":{\"magnitude\":3494.4106433,\"unit\":28}},\"compensated\":{\"mathematicalModels\":{\"MM0123\":{\"pressure\":{\"output\":{\"magnitude\":0.270032,\"unit\":3},\"error\":{\"magnitude\":0.011704121,\"unit\":7}},\"temperature\":{\"output\":{\"magnitude\":19.5338,\"unit\":4},\"error\":{\"magnitude\":-0.017083039,\"unit\":4}}}}}},{\"reference\":\"F_12300_XX_0000098765\",\"environmentTarget\":{\"pressure\":{\"magnitude\":0.35,\"unit\":3},\"temperature\":{\"magnitude\":20.0,\"unit\":4}},\"environment\":{\"pressure\":{\"magnitude\":0.350009,\"unit\":3},\"temperature\":{\"magnitude\":19.5509,\"unit\":4},\"supply\":{\"magnitude\":1.0,\"unit\":18}},\"raw\":{\"signal\":{\"magnitude\":64.987586352,\"unit\":22},\"bridgeResistance\":{\"magnitude\":3490.0811649,\"unit\":28}},\"compensated\":{\"mathematicalModels\":{\"MM0123\":{\"pressure\":{\"output\":{\"magnitude\":0.350011,\"unit\":3},\"error\":{\"magnitude\":0.00046731692,\"unit\":7}},\"temperature\":{\"output\":{\"magnitude\":19.5336,\"unit\":4},\"error\":{\"magnitude\":-0.017292929,\"unit\":4}}}}}},{\"reference\":\"F_12300_XX_0000098765\",\"environmentTarget\":{\"pressure\":{\"magnitude\":0.03,\"unit\":3},\"temperature\":{\"magnitude\":40.0,\"unit\":4}},\"environment\":{\"pressure\":{\"magnitude\":0.0299991,\"unit\":3},\"temperature\":{\"magnitude\":39.7284,\"unit\":4},\"supply\":{\"magnitude\":1.0,\"unit\":18}},\"raw\":{\"signal\":{\"magnitude\":18.24225896,\"unit\":22},\"bridgeResistance\":{\"magnitude\":3684.2373732,\"unit\":28}},\"compensated\":{\"mathematicalModels\":{\"MM0123\":{\"pressure\":{\"output\":{\"magnitude\":0.0300144,\"unit\":3},\"error\":{\"magnitude\":0.0043610692,\"unit\":7}},\"temperature\":{\"output\":{\"magnitude\":39.721,\"unit\":4},\"error\":{\"magnitude\":-0.0074241742,\"unit\":4}}}}}},{\"reference\":\"F_12300_XX_0000098765\",\"environmentTarget\":{\"pressure\":{\"magnitude\":0.11,\"unit\":3},\"temperature\":{\"magnitude\":40.0,\"unit\":4}},\"environment\":{\"pressure\":{\"magnitude\":0.110014,\"unit\":3},\"temperature\":{\"magnitude\":39.7284,\"unit\":4},\"supply\":{\"magnitude\":1.0,\"unit\":18}},\"raw\":{\"signal\":{\"magnitude\":30.319780069,\"unit\":22},\"bridgeResistance\":{\"magnitude\":3679.6145564,\"unit\":28}},\"compensated\":{\"mathematicalModels\":{\"MM0123\":{\"pressure\":{\"output\":{\"magnitude\":0.109978,\"unit\":3},\"error\":{\"magnitude\":-0.010241732,\"unit\":7}},\"temperature\":{\"output\":{\"magnitude\":39.7212,\"unit\":4},\"error\":{\"magnitude\":-0.0072277104,\"unit\":4}}}}}},{\"reference\":\"F_12300_XX_0000098765\",\"environmentTarget\":{\"pressure\":{\"magnitude\":0.19,\"unit\":3},\"temperature\":{\"magnitude\":40.0,\"unit\":4}},\"environment\":{\"pressure\":{\"magnitude\":0.190005,\"unit\":3},\"temperature\":{\"magnitude\":39.7284,\"unit\":4},\"supply\":{\"magnitude\":1.0,\"unit\":18}},\"raw\":{\"signal\":{\"magnitude\":42.36485294,\"unit\":22},\"bridgeResistance\":{\"magnitude\":3675.0275052,\"unit\":28}},\"compensated\":{\"mathematicalModels\":{\"MM0123\":{\"pressure\":{\"output\":{\"magnitude\":0.190005,\"unit\":3},\"error\":{\"magnitude\":-7.050573E-05,\"unit\":7}},\"temperature\":{\"output\":{\"magnitude\":39.7176,\"unit\":4},\"error\":{\"magnitude\":-0.01080946,\"unit\":4}}}}}},{\"reference\":\"F_12300_XX_0000098765\",\"environmentTarget\":{\"pressure\":{\"magnitude\":0.27,\"unit\":3},\"temperature\":{\"magnitude\":40.0,\"unit\":4}},\"environment\":{\"pressure\":{\"magnitude\":0.26999,\"unit\":3},\"temperature\":{\"magnitude\":39.7284,\"unit\":4},\"supply\":{\"magnitude\":1.0,\"unit\":18}},\"raw\":{\"signal\":{\"magnitude\":54.36493409,\"unit\":22},\"bridgeResistance\":{\"magnitude\":3670.551534,\"unit\":28}},\"compensated\":{\"mathematicalModels\":{\"MM0123\":{\"pressure\":{\"output\":{\"magnitude\":0.270008,\"unit\":3},\"error\":{\"magnitude\":0.0050316864,\"unit\":7}},\"temperature\":{\"output\":{\"magnitude\":39.7178,\"unit\":4},\"error\":{\"magnitude\":-0.010603724,\"unit\":4}}}}}},{\"reference\":\"F_12300_XX_0000098765\",\"environmentTarget\":{\"pressure\":{\"magnitude\":0.35,\"unit\":3},\"temperature\":{\"magnitude\":40.0,\"unit\":4}},\"environment\":{\"pressure\":{\"magnitude\":0.350002,\"unit\":3},\"temperature\":{\"magnitude\":39.7284,\"unit\":4},\"supply\":{\"magnitude\":1.0,\"unit\":18}},\"raw\":{\"signal\":{\"magnitude\":66.318186077,\"unit\":22},\"bridgeResistance\":{\"magnitude\":3666.1189358,\"unit\":28}},\"compensated\":{\"mathematicalModels\":{\"MM0123\":{\"pressure\":{\"output\":{\"magnitude\":0.349977,\"unit\":3},\"error\":{\"magnitude\":-0.0071103905,\"unit\":7}},\"temperature\":{\"output\":{\"magnitude\":39.7143,\"unit\":4},\"error\":{\"magnitude\":-0.01416877,\"unit\":4}}}}}},{\"reference\":\"F_12300_XX_0000098765\",\"environmentTarget\":{\"pressure\":{\"magnitude\":0.03,\"unit\":3},\"temperature\":{\"magnitude\":60.0,\"unit\":4}},\"environment\":{\"pressure\":{\"magnitude\":0.0299987,\"unit\":3},\"temperature\":{\"magnitude\":59.8651,\"unit\":4},\"supply\":{\"magnitude\":1.0,\"unit\":18}},\"raw\":{\"signal\":{\"magnitude\":19.430746391,\"unit\":22},\"bridgeResistance\":{\"magnitude\":3876.8980666,\"unit\":28}},\"compensated\":{\"mathematicalModels\":{\"MM0123\":{\"pressure\":{\"output\":{\"magnitude\":0.030018,\"unit\":3},\"error\":{\"magnitude\":0.0055081768,\"unit\":7}},\"temperature\":{\"output\":{\"magnitude\":59.9331,\"unit\":4},\"error\":{\"magnitude\":0.067989781,\"unit\":4}}}}}},{\"reference\":\"F_12300_XX_0000098765\",\"environmentTarget\":{\"pressure\":{\"magnitude\":0.11,\"unit\":3},\"temperature\":{\"magnitude\":60.0,\"unit\":4}},\"environment\":{\"pressure\":{\"magnitude\":0.109998,\"unit\":3},\"temperature\":{\"magnitude\":59.8651,\"unit\":4},\"supply\":{\"magnitude\":1.0,\"unit\":18}},\"raw\":{\"signal\":{\"magnitude\":31.601420575,\"unit\":22},\"bridgeResistance\":{\"magnitude\":3872.2133853,\"unit\":28}},\"compensated\":{\"mathematicalModels\":{\"MM0123\":{\"pressure\":{\"output\":{\"magnitude\":0.10996,\"unit\":3},\"error\":{\"magnitude\":-0.010962099,\"unit\":7}},\"temperature\":{\"output\":{\"magnitude\":59.9359,\"unit\":4},\"error\":{\"magnitude\":0.070771131,\"unit\":4}}}}}},{\"reference\":\"F_12300_XX_0000098765\",\"environmentTarget\":{\"pressure\":{\"magnitude\":0.19,\"unit\":3},\"temperature\":{\"magnitude\":60.0,\"unit\":4}},\"environment\":{\"pressure\":{\"magnitude\":0.189992,\"unit\":3},\"temperature\":{\"magnitude\":59.8651,\"unit\":4},\"supply\":{\"magnitude\":1.0,\"unit\":18}},\"raw\":{\"signal\":{\"magnitude\":43.750703619,\"unit\":22},\"bridgeResistance\":{\"magnitude\":3867.5737968,\"unit\":28}},\"compensated\":{\"mathematicalModels\":{\"MM0123\":{\"pressure\":{\"output\":{\"magnitude\":0.190001,\"unit\":3},\"error\":{\"magnitude\":0.0027007716,\"unit\":7}},\"temperature\":{\"output\":{\"magnitude\":59.9377,\"unit\":4},\"error\":
